vi "MRate Interpolation (FPGA).vi"   [LabVIEW 2023]
uses:
  <vilib>/eio/EIONode/EIONode.xnode
  <vilib>/rvi/DataTransferAndStorage/Container/XNode/niFpgaContainer.xnode
  <vilib>/rvi/eio/common/nirviEmuTemplateMethod_errors.vi
  <vilib>/rvi/FIFO/Fifo_Resource/nirvififoEmulationWrite.vi
  <vilib>/rvi/FIFO/Fifo_Resource/nirvififoEmulationRead.vi
  <vilib>/rvi/interface/RandomDataEmulation/nirviRandomDataFpgaReadWriteTemplate.vi
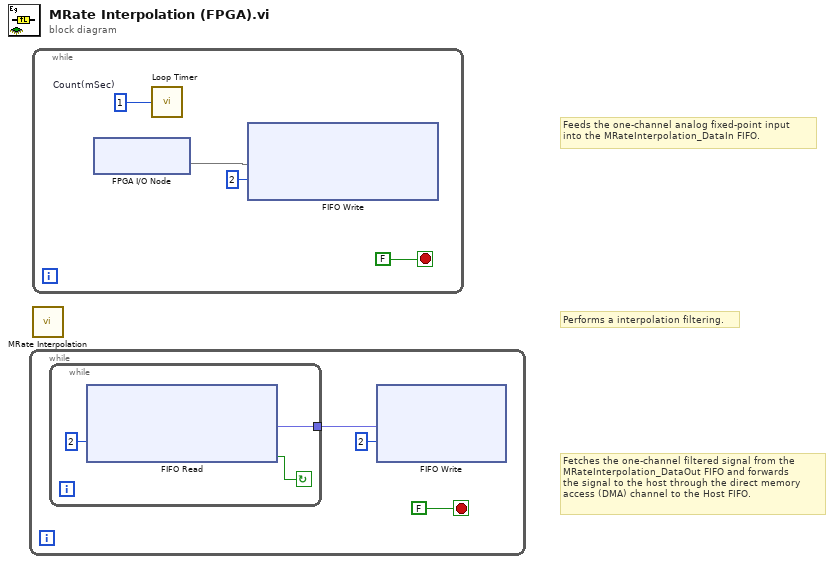
[diagram p0: block diagram]
diagram:
  # "Fetches the one-channel filtered signal from the \nMRateInterpolation_DataOut FIFO and forwards \nthe signal to the host through the direct memory \naccess (DMA) channel to the Host FIFO."
  # "Feeds the one-channel analog fixed-point input\ninto the MRateInterpolation_DataIn FIFO."
  # "Performs a interpolation filtering."
  n1 = while {
    stop <- FALSE stop-if-true
    n2 = while {
      tunnel: [w4] -> w1
      stop <- w5 continue-if-true
      n3 = xnode ("FIFO Read")("Timeout"=2) -> ("Element"=w4:fxp<+/-,32,7>, "Timed Out?"=w5:bool)  [unwired: 1 in, 1 out]
    }
    n4 = xnode ("FIFO Write")("Element"=w1, "Timeout"=2) -> ()  [unwired: 1 in, 2 out]
  }
  n5 = while {
    stop <- FALSE stop-if-true
    w9 = u16 1  # Count(mSec)
    n6 = xnode "FPGA I/O Node"() -> ("Mod1/AI0"=w8)  [unwired: 1 in, 1 out]
    n7 = call "Loop Timer"("Count(uSec)"=w9) -> ()  [unwired: 1 out]
    n8 = xnode ("FIFO Write")("Element"=w8, "Timeout"=2) -> ()  [unwired: 1 in, 2 out]
  }
  n9 = call "MRate Interpolation.vi"() -> ()  [unwired: 1 out]
